vi "ExitingState.vi"(0 "StateIn":T7 {"ILoad" format="%_6g"; "Fault Registers" format="%016x"; "VLoad" format="%_6g"; "VDCLink" format="%_6g"; "Detected Frequency" format="%1_6g"}, 1 "Interfaces":T1, 5 "ExitingState":T6, 11 "error in (no error)":errorcluster) -> (4 "StateOut":T7 {"ILoad" format="%_6g"; "Fault Registers" format="%016x"; "VLoad" format="%_6g"; "VDCLink" format="%_6g"; "Detected Frequency" format="%1_6g"}, 15 "error out":errorcluster)   [LabVIEW 2017, in "AppStateMachine runtime.lvclass"]
uses:
  AppStateMachine runtime.lvclass
  State.ctl
  StateId.ctl
  LED_Color.ctl
  Interfaces.ctl
  <vilib>/NI/NI JSONRPC Server Framework/Classes/Server/JSONRPC Server.lvclass
  <instrlib>/_niInstr/Instruction Framework/v1/Host/Instruction Target/niInstr Instruction Target v1 Host.lvclass
  <instrlib>/_niInstr/Instruction Framework/v1/Host/Instruction Framework Context/niInstr Instruction Framework Context v1 Host.lvclass
  FPGA/FPGAtypedef.ctl
  <vilib>/NI/PowerElectronicsControl/ThreePhasePLL/Interface/InterfaceRef.ctl
  <vilib>/NI/PowerElectronicsControl/ActiveFrontEnd/AFE_Interface/InterfaceRef.ctl
  <vilib>/NI/PowerElectronicsControl/Buck-Boost/RealTime/Interface.ctl
  <vilib>/Utility/error.llb/Error Cluster From Error Code.vi
  <vilib>/rvi/errors/niLvFpgaAdjustHostInterfaceError.vi
  <vilib>/rvi/interface/nirviReadWriteControl/nirviReadWriteControl.xnode
  NiFpgaLv.dll
  <vilib>/rvi/interface/Simulation/niFpgaSimulationCallBeginRW.vi
  <vilib>/NI/PowerElectronicsControl/Buck-Boost/RealTime/BuckBoostInterface.lvlib
  <vilib>/NI/PowerElectronicsControl/ThreePhasePLL/Interface/ThreePhasePLLInterface.lvlib
  <vilib>/NI/PowerElectronicsControl/ActiveFrontEnd/AFE_Interface/AFE_interface.lvlib
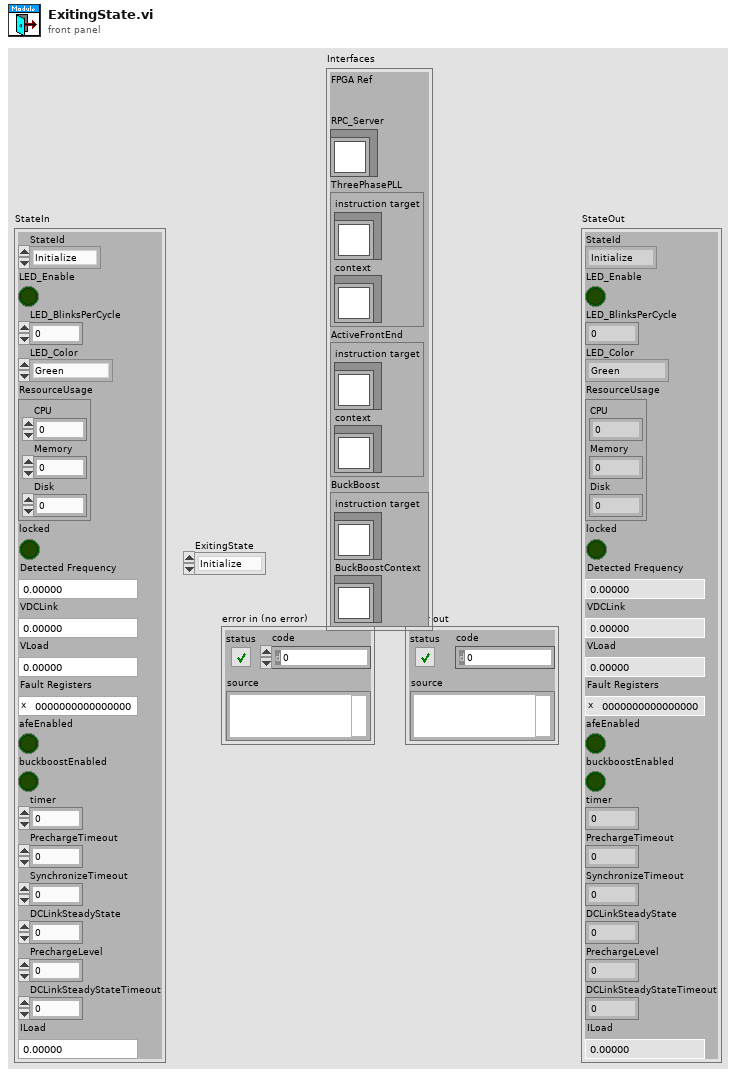
[diagram p1: front panel]
types:
  T1 = typedef "AppStateMachine runtime.lvclass/Interfaces.ctl" = cluster{"FPGA Ref":T2, "RPC_Server":refnum<class "JSONRPC Server.lvclass">, "ThreePhasePLL":T3, "ActiveFrontEnd":T4, "BuckBoost":T5}
  T2 = typedef "AppStateMachine runtime.lvclass/FPGAtypedef.ctl" = refnum<k20>
  T3 = typedef "ThreePhasePLLInterface.lvlib/InterfaceRef.ctl" = cluster{"instruction target":refnum<class "niInstr Instruction Target v1 Host.lvclass">, "context":refnum<class "niInstr Instruction Framework Context v1 Host.lvclass">}
  T4 = typedef "AFE_interface.lvlib/InterfaceRef.ctl" = cluster{"instruction target":refnum<class "niInstr Instruction Target v1 Host.lvclass">, "context":refnum<class "niInstr Instruction Framework Context v1 Host.lvclass">}
  T5 = typedef "BuckBoostInterface.lvlib/Interface.ctl" = cluster{"instruction target":refnum<class "niInstr Instruction Target v1 Host.lvclass">, "BuckBoostContext":refnum<class "niInstr Instruction Framework Context v1 Host.lvclass">}
  T6 = typedef "AppStateMachine runtime.lvclass/StateId.ctl" = enum16{"Initialize", "Idle", "TunePLL", "TuneAFE", "TuneBuckBoost", "Precharge", "Synchronize", "Ready", "EnableAFE", "EnableBuckBoost", "Powered", "SafeState", "UnrecoverableSafeState"}
  T7 = typedef "AppStateMachine runtime.lvclass/State.ctl" = cluster{"StateId":T6, "LED_Enable":bool, "LED_BlinksPerCycle":i32, "LED_Color":T8, "ResourceUsage":cluster{"CPU":dbl, "Memory":dbl, "Disk":dbl}, "locked":bool, "Detected Frequency":dbl, "VDCLink":dbl, "VLoad":dbl, "Fault Registers":u64, "afeEnabled":bool, "buckboostEnabled":bool, "timer":u32, "PrechargeTimeout":u32, "SynchronizeTimeout":u32, "DCLinkSteadyState":dbl, "PrechargeLevel":dbl, "DCLinkSteadyStateTimeout":u32, "ILoad":dbl}
  T8 = typedef "AppStateMachine runtime.lvclass/LED_Color.ctl" = enum16{"Green", "Yellow"}
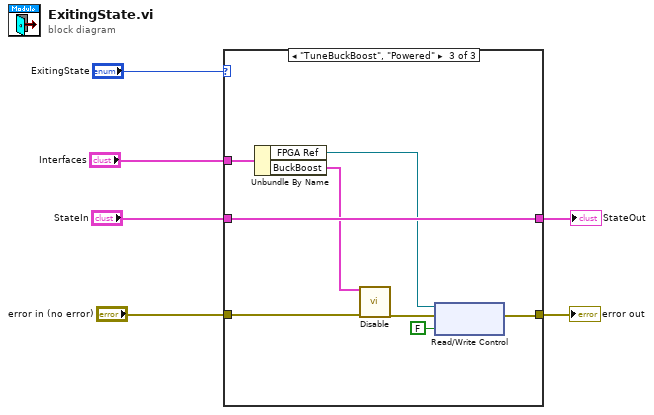
[diagram p0: block diagram]
diagram:
  n1 = case shown="\"TuneBuckBoost\", \"Powered\"" "ExitingState" {
    tunnel: "error in (no error)" -> [w8 w10 w12]
    tunnel: [w8 w10 w16] -> w6
    tunnel: "Interfaces" -> [_ _ w17]
    tunnel: "StateIn" -> [w7 w9 w18]
    tunnel: [w7 w9 w18] -> w2
    frame Default {
    }
    frame "Idle" {
    }
    frame "TuneBuckBoost", "Powered" {
      n2 = Unbundle By Name(w17) -> ("FPGA Ref"=w15:T2, "BuckBoost"=w11:T5)
      n3 = call <vilib>:"Disable.vi"("Interface in"=w11, "error in (no error)"=w12) -> ("error out"=w13:errorcluster)  [unwired: 12 in, 1 out]
      n4 = xnode "Read/Write Control"("FPGA VI Reference In"=w15, "error in"=w13, "enableAFE"=FALSE) -> ("error out"=w16:errorcluster)  [unwired: 1 out]
    }
  }
  "error out" <- w6
  "StateOut" <- w2
